vi "tester.vi"() -> ()   [LabVIEW 2010]
uses:
  magic ring.xctl
panel:
  out "String":string
  in  "magic ring":string(xcontrol)
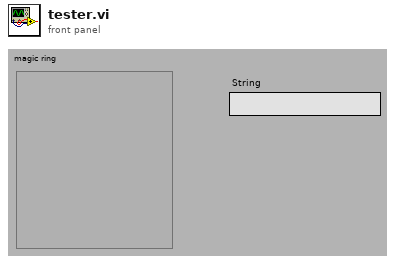
[diagram p1: front panel]
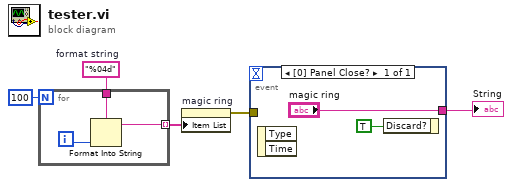
[diagram p0: block diagram]
diagram:
  w2 = "%04d"  # format string
  n1 = for {
    N: 100 -> [_]
    tunnel: [w7] -> w4 mode=indexing
    tunnel: w2 -> [w6]
    i -> [w8]
    n2 = Format Into String(format string=w6, w8) -> (resulting string=w7:string)  [unwired: 2 in, 1 out]
  }
  n3 = property on="magic ring" class="magic ring (strict)"("Item List"=w4) -> (error out=w3:errorcluster)  [unwired: 2 in, 1 out]
  n4 = event shown="[0] Panel Close?" {
    selector: _ -> [_]
    dyn-events: _ -> [_]
    timeout: _ -> [_]
    tunnel: w3 -> [_]
    tunnel: ["magic ring"] -> w1
    event Panel Close? {
      n5 = event-data() -> ()  [unwired: 1 in, 2 out]
      n6 = event-data("Discard?"=TRUE) -> ()  [unwired: 1 in, 1 out]
    }
  }
  "String" <- w1
